vi "GrowArray.vi"(9 "grow":i32, 10 "index":i32, 11 "SubChannel in":refnum<class "SubChannelCPU.lvclass">) -> (3 "SubChannel out":refnum<class "SubChannelCPU.lvclass">)   [LabVIEW 2019, in "MessengerM.lvlib" / "SubChannelCPU.lvclass"]
uses:
  SubChannelCPU.lvclass
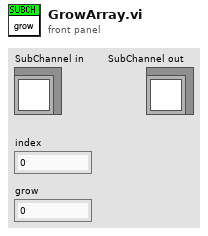
[diagram p1: front panel]
types:
  T1 = typedef "MessengerM.lvlib/Element.ctl" = string
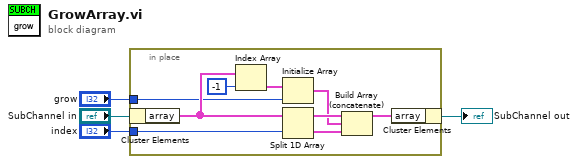
[diagram p0: block diagram]
diagram:
  n1 = in-place {
    in-place-border: "index" -> [w12]
    in-place-border: "grow" -> [w10]
    n2 = in-place-cluster #1("SubChannel in") -> ("array"=w13:cluster{"elt":T1}[])
    n3 = Index Array(array=w13, index=-1) -> (element=w6:cluster{"elt":T1})
    n4 = Initialize Array(w6, w10) -> (w5:cluster{"elt":T1}[])
    n5 = Split 1D Array(array=w13, index=w12) -> (first subarray=w9:cluster{"elt":T1}[], second subarray=w8:cluster{"elt":T1}[])
    n6 = Build Array (concatenate)(w9, w5, w8) -> (w11:cluster{"elt":T1}[])
    n7 = in-place-cluster #1("array"=w11) -> (→"SubChannel out":refnum<class "SubChannelCPU.lvclass">)
  }
